vi "Change Temperature V2.00.vi"(4 "error in":errorcluster, 6 "Rat(dlogR/dlogT)":dbl=0.66 format="%.2f", 7 "TempControl":bool[](array[boolean]), 8 "Current Field":dbl=9.0 format="%.2f", 9 "Temp Tolerance":dbl format="%.2f", 10 "Desired Temperature":dbl=305.0 format="%.2f", 11 "GPIB Address":u16=15 min=2 max=31 step=1) -> (0 "error out":errorcluster, 3 "Final Temp":dbl format="%.2f")   [LabVIEW 2024]
uses:
  Globals and TypeDefs/Type Definitions.llb/3 way Status.ctl
  Globals and TypeDefs/Global Varibal Control.vi
  Globals and TypeDefs/gStatus.vi
panel:
  # "Temperature Controller Controls"
  # "Exist?"
  # "TC Enable or Monitor"
  # "Magneto-Correction?"
  # "Auto-Advancing?"
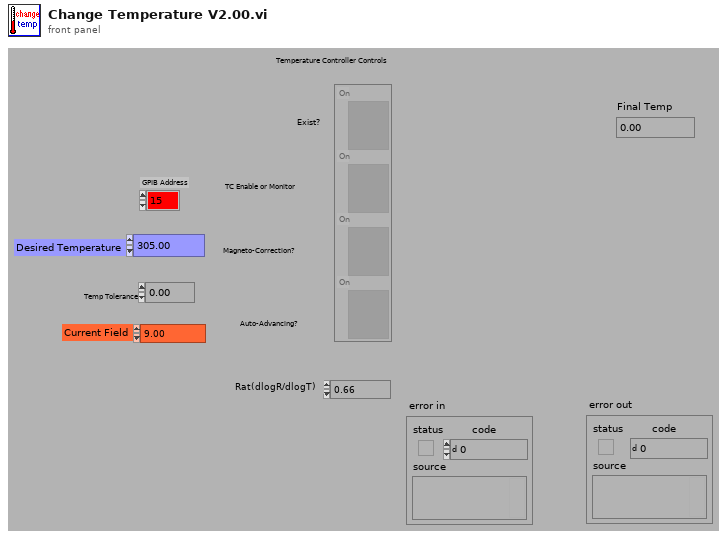
[diagram p1: front panel]
types:
  T1 = typedef "3 way Status.ctl" = u8
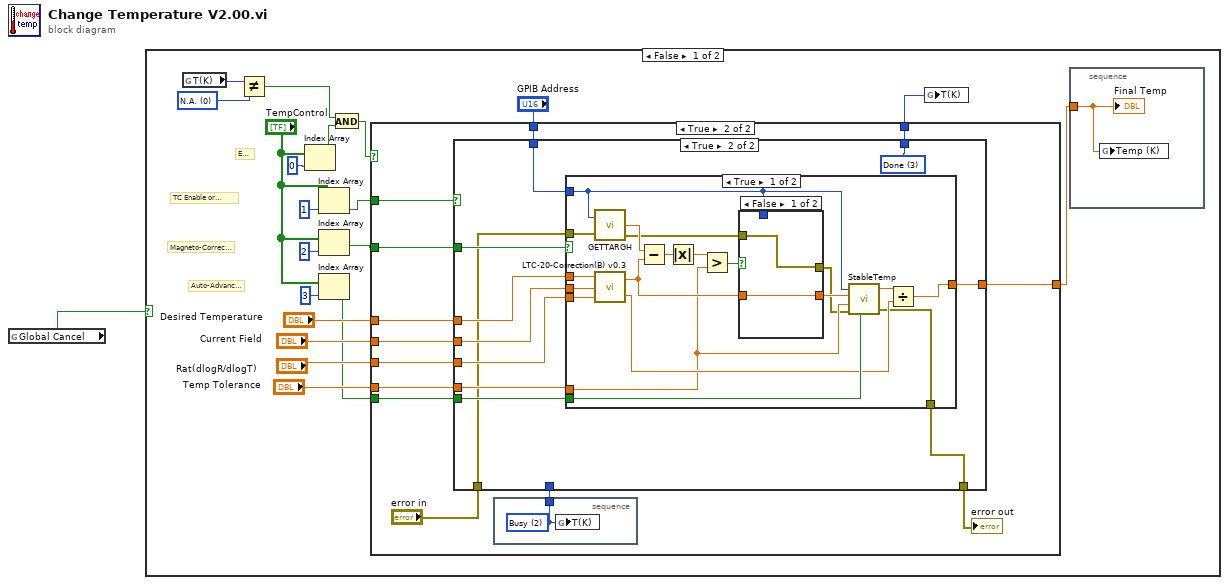
[diagram p0: block diagram]
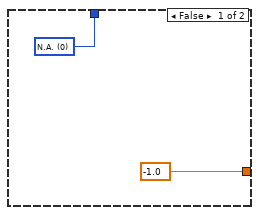
[diagram p2: hidden frame]
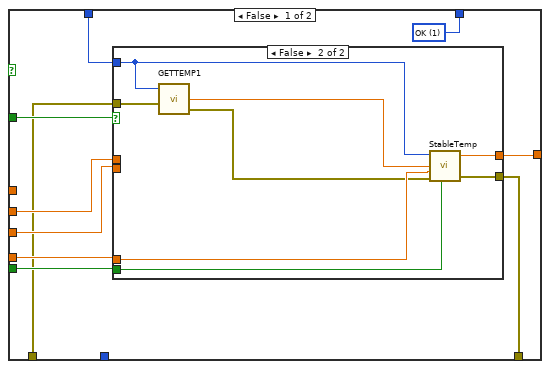
[diagram p3: hidden frame]
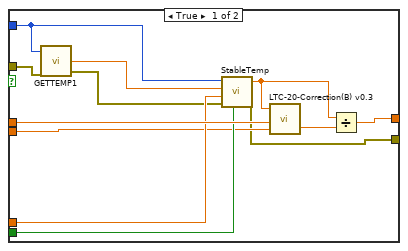
[diagram p4: hidden frame]
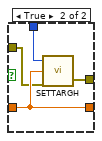
[diagram p5: hidden frame]
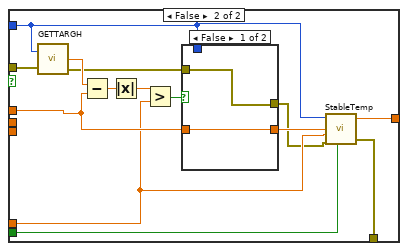
[diagram p6: hidden frame]
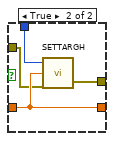
[diagram p7: hidden frame]
diagram:
  n1 = global read "Global Varibal Control.vi" "Global Cancel"() -> (w1:bool)
  n2 = case shown="False" w1 {
    frame False {
      w6 = T1 0 items=["N.A.", "OK", "Busy", "Done"] ("y")
      # "Exist?"
      # "Auto-Advancing?"
      # "Magneto-Correction?"
      # "TC Enable or Monitor"
      n3 = global read "gStatus.vi" "T(K)"() -> (w7:T1)
      n4 = Not Equal?(x=w7, y=w6) -> (x != y?=w3:bool)
      n5 = Index Array(array="TempControl", index=0) -> (element=w5:bool)
      n6 = Index Array(array="TempControl", index=1) -> (element=w16:bool)
      n7 = Index Array(array="TempControl", index=2) -> (element=w11:bool)
      n8 = Index Array(array="TempControl", index=3) -> (element=w9:bool)
      n9 = And(x=w3, y=w5) -> (x .and. y?=w4:bool)
      n10 = case shown="True" w4 {
        tunnel: w16 -> [_ w37]
        tunnel: "Desired Temperature" -> [_ w36]
        tunnel: "Current Field" -> [_ w35]
        tunnel: "Rat(dlogR/dlogT)" -> [_ w34]
        tunnel: "GPIB Address" -> [_ w33]
        tunnel: w11 -> [_ w32]
        tunnel: "Temp Tolerance" -> [_ w31]
        tunnel: w9 -> [_ w30]
        tunnel: [-1.0 ("Final Temp") w29] -> w8
        tunnel: [w23 w26] -> w2
        frame False {
          w23 = T1 0 items=["N.A.", "OK", "Busy", "Done"] ("y")
        }
        frame True {
          n11 = stacked-sequence {
            tunnel: [w38] -> w25
            frame #0 {
              w38 = T1 2 items=["N.A.", "OK", "Busy", "Done"] ("T(K)")
              n12 = global write "gStatus.vi" "T(K)"(w38) -> ()
            }
          }
          n13 = case shown="True" w37 {
            tunnel: w36 -> [_ w79]
            tunnel: w35 -> [w46 w78]
            tunnel: w34 -> [w45 w77]
            tunnel: w33 -> [w47 w76]
            tunnel: w32 -> [w48 w75]
            tunnel: w31 -> [w43 w74]
            tunnel: w30 -> [w44 w73]
            tunnel: [w42 w72] -> w29
            tunnel: "error in" -> [w41 w71]
            tunnel: [w40 w70] -> w27
            tunnel: [w39 w69] -> w26
            tunnel: w25 -> [_ _]
            frame False {
              w39 = T1 1 items=["N.A.", "OK", "Busy", "Done"] ("T(K)")
              n14 = case shown="False" w48 {
                tunnel: w46 -> [w60 _]
                tunnel: w45 -> [w54 _]
                tunnel: w47 -> [w55 w65]
                tunnel: w43 -> [w59 w66]
                tunnel: w44 -> [w58 w68]
                tunnel: [w56 w67] -> w42
                tunnel: w41 -> [w51 w63]
                tunnel: [w49 w61] -> w40
                frame True {
                  n15 = call "GETTEMP1.VI"("GPIB Device"=w55, "error in (no error)"=w51) -> ("Sensor 1"=w53:sgl, "error out"=w50:errorcluster)  [unwired: 1 out]
                  n16 = call "StableTemp.VI"("GPIB Device"=w55, "Desired Temp"=w53, "Tolerance"=w59, "error in (no error)"=w50, "AutoAdvancing"=w58) -> ("Final Temp"=w52:sgl, "error out"=w49:errorcluster)  [unwired: 1 in]
                  n17 = call "LTC-20-Correction(B) v0.3.vi"("Rat(dlogR/dlogT)"=w54, "Current Field"=w60, "Desired Temperature"=w52) -> ("Correction Coef."=w57:dbl)  [unwired: 1 out]
                  n18 = Divide(x=w52, y=w57) -> (x/y=w56:dbl)
                }
                frame False {
                  n19 = call "GETTEMP1.VI"("GPIB Device"=w65, "error in (no error)"=w63) -> ("Sensor 1"=w64:sgl, "error out"=w62:errorcluster)  [unwired: 1 out]
                  n20 = call "StableTemp.VI"("GPIB Device"=w65, "Desired Temp"=w64, "Tolerance"=w66, "error in (no error)"=w62, "AutoAdvancing"=w68) -> ("Final Temp"=w67:sgl, "error out"=w61:errorcluster)  [unwired: 1 in]
                }
              }
            }
            frame True {
              w69 = T1 3 items=["N.A.", "OK", "Busy", "Done"] ("T(K)")
              n21 = case shown="True" w75 {
                tunnel: w79 -> [w98 w115]
                tunnel: w78 -> [w97 _]
                tunnel: w77 -> [w96 _]
                tunnel: w76 -> [w89 w113]
                tunnel: w74 -> [w82 w110]
                tunnel: w73 -> [w88 w112]
                tunnel: [w85 w109] -> w72
                tunnel: w71 -> [w84 w108]
                tunnel: [w80 w105] -> w70
                frame True {
                  n22 = call "GETTARGH.vi"("GPIB Device"=w89, "error in (no error)"=w84) -> ("Heater Setpoint"=w91:sgl, "error out"=w83:errorcluster)  [unwired: 1 out]
                  n23 = call "LTC-20-Correction(B) v0.3.vi"("Rat(dlogR/dlogT)"=w96, "Current Field"=w97, "Desired Temperature"=w98) -> ("Correction Coef."=w86:dbl, "TempSetpoint"=w92:dbl)
                  n24 = Subtract(x=w91, y=w92) -> (x-y=w95:dbl)
                  n25 = Absolute Value(x=w95) -> (abs(x)=w94:dbl)
                  n26 = Greater?(x=w94, y=w82) -> (0:w93:bool)
                  n27 = case shown="False" w93 {
                    tunnel: w92 -> [w100 w103]
                    tunnel: w89 -> [_ w104]
                    tunnel: [w100 w103] -> w90
                    tunnel: w83 -> [w99 w102]
                    tunnel: [w99 w101] -> w81
                    frame False {
                    }
                    frame True {
                      n28 = call "SETTARGH.vi"("error in (no error)"=w102, "Heater Setpoint"=w103, "GPIB Device"=w104) -> ("error out"=w101:errorcluster)  [unwired: 1 out]
                    }
                  }
                  n29 = call "StableTemp.VI"("GPIB Device"=w89, "Desired Temp"=w90, "Tolerance"=w82, "error in (no error)"=w81, "AutoAdvancing"=w88) -> ("Final Temp"=w87:sgl, "error out"=w80:errorcluster)  [unwired: 1 in]
                  n30 = Divide(x=w87, y=w86) -> (x/y=w85:dbl)
                }
                frame False {
                  n31 = call "GETTARGH.vi"("GPIB Device"=w113, "error in (no error)"=w108) -> ("Heater Setpoint"=w114:sgl, "error out"=w107:errorcluster)  [unwired: 1 out]
                  n32 = Subtract(x=w114, y=w115) -> (x-y=w118:dbl)
                  n33 = Absolute Value(x=w118) -> (abs(x)=w117:dbl)
                  n34 = Greater?(x=w117, y=w110) -> (0:w116:bool)
                  n35 = case shown="False" w116 {
                    tunnel: w115 -> [w120 w123]
                    tunnel: w113 -> [_ w124]
                    tunnel: [w120 w123] -> w111
                    tunnel: w107 -> [w119 w122]
                    tunnel: [w119 w121] -> w106
                    frame False {
                    }
                    frame True {
                      n36 = call "SETTARGH.vi"("error in (no error)"=w122, "Heater Setpoint"=w123, "GPIB Device"=w124) -> ("error out"=w121:errorcluster)  [unwired: 1 out]
                    }
                  }
                  n37 = call "StableTemp.VI"("GPIB Device"=w113, "Desired Temp"=w111, "Tolerance"=w110, "error in (no error)"=w106, "AutoAdvancing"=w112) -> ("Final Temp"=w109:sgl, "error out"=w105:errorcluster)  [unwired: 1 in]
                }
              }
            }
          }
          "error out" <- w27
        }
      }
      n38 = global write "gStatus.vi" "T(K)"(w2) -> ()
      n39 = stacked-sequence {
        tunnel: w8 -> [w22]
        frame #0 {
          n40 = global write "Global Varibal Control.vi" "Temp (K)"(w22) -> ()
          "Final Temp" <- w22
        }
      }
    }
    frame True {
    }
  }
